vi "DSF.Engine.Memory.Buffer.Errors.vi"   [LabVIEW 2016, in "DSF.Engine.lvlib" / "DSF.Engine.Memory.Buffer.lvclass"]
uses:
  DSF.Engine.Memory.Buffer.lvclass
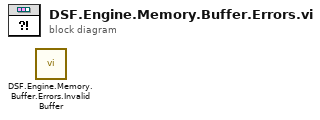
[diagram p0: block diagram]
diagram:
  n1 = call "DSF.Engine.Memory.Buffer.Errors.Invalid Buffer.vi"() -> ()  [unwired: 10 in, 2 out]
